vi "Transfer Offsets.vi"(1 "error in":errorcluster) -> (0 "error out":errorcluster)   [LabVIEW 2009]
uses:
  Data Access Objects/Metadata/DAO Actions.ctl
  Global Data/Dataset Transaction Id.ctl
  Global Data/Dataset Source.ctl
  Global Data/Dataset Type.ctl
  Apps/Yes No Button.ctl
  Data Access Objects/Metadata/LBCB Number.ctl
  Control Loop/LBCB_Conversions_Actions.ctl
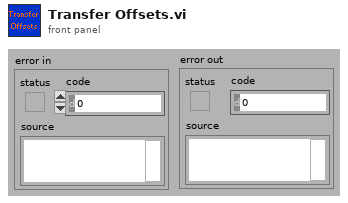
[diagram p1: front panel]
types:
  T1 = typedef "Dataset Type.ctl" = enum16{"LVDT", "Load Cell", "Actuator Command", "Servo Error", "Displacement Command", "Displacement", "Force"}
  T2 = typedef "LBCB Number.ctl" = enum16{"LBCB1", "LBCB2"}
  T3 = typedef "Dataset Source.ctl" = enum16{"LBCB 1", "LBCB 2", "Combined", "External Sensors"}
  T4 = typedef "Dataset Transaction Id.ctl" = cluster{"Dataset Source":T3, "Dataset Type":T1, "Hold":T5, "Volts":T5, "Tag":string}
  T5 = typedef "Yes No Button.ctl" = bool
  T6 = typedef "DAO Actions.ctl" = enum16{"Init", "Get", "Set"}
  T7 = typedef "LBCB Position.ctl" = cluster{"Motion Center":dbl[], "Transformation Matrix":dbl[][]}
  T8 = typedef "LBCB Settings.ctl" = cluster{"Size":T9, "Type":T10}
  T9 = typedef "LBCB Size.ctl" = enum16{"1/5th-scale LBCB", "Full-scale LBCB", "Portable LBCB"}
  T10 = typedef "LBCB Type.ctl" = enum16{"X Actuators On The Left", "X Actuators On The Right"}
  T11 = typedef "LBCB_Conversions_Actions.ctl" = enum16{"A2C", "C2A", "Set Log Filename", "Init"}
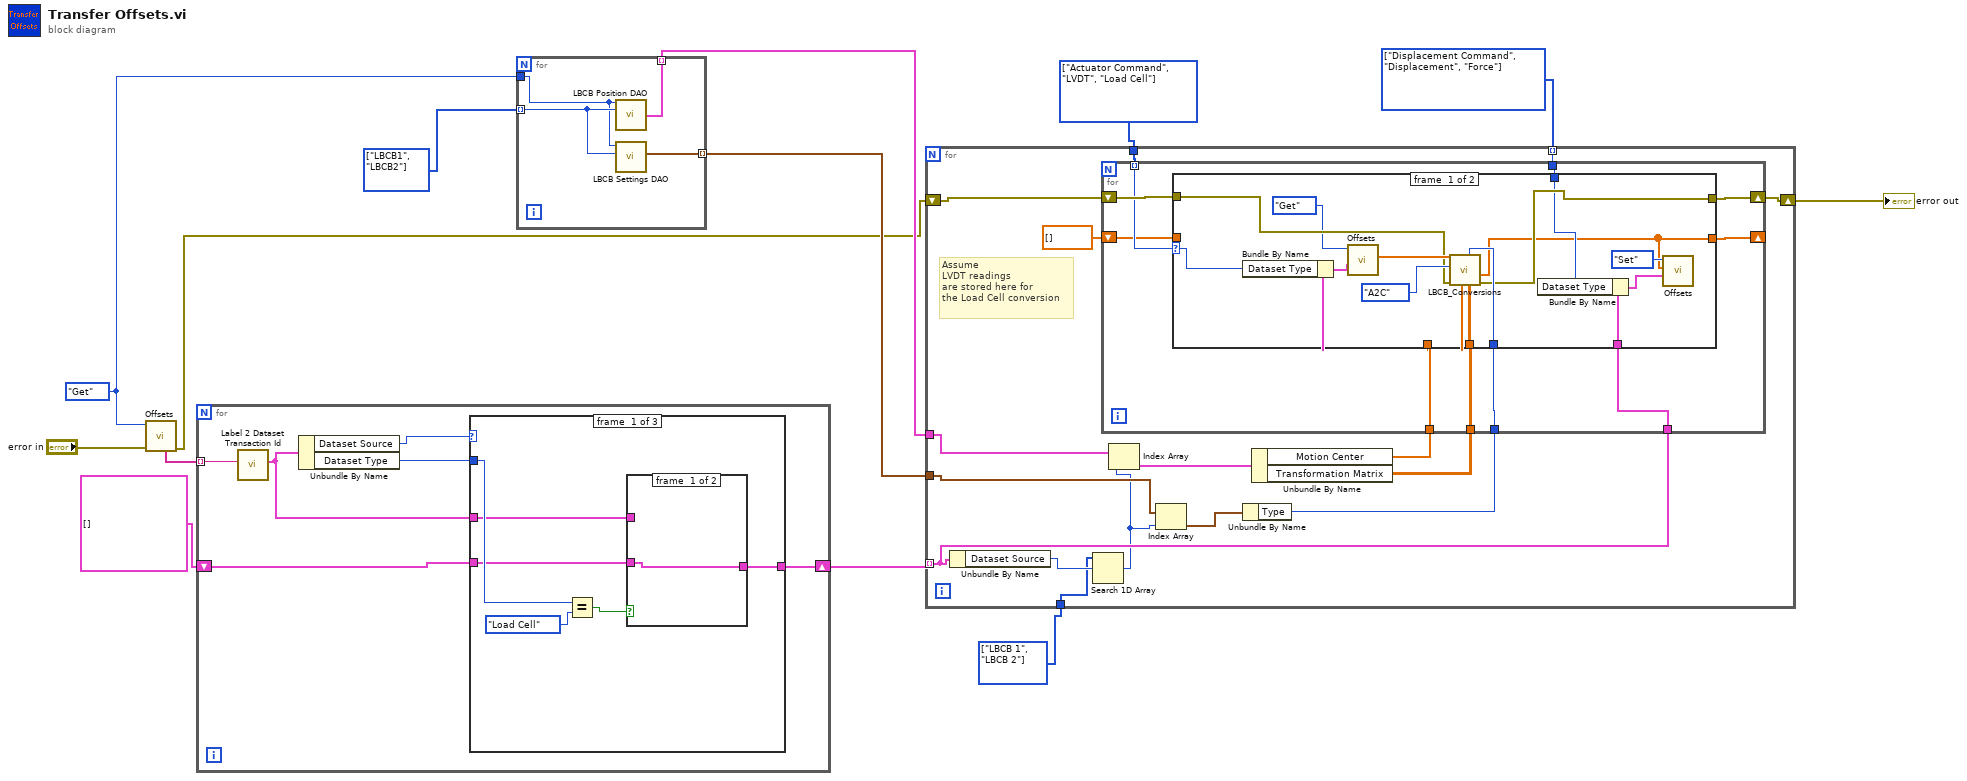
[diagram p0: block diagram]
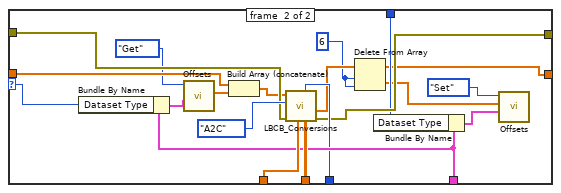
[diagram p2: hidden frame]
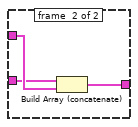
[diagram p3: hidden frame]
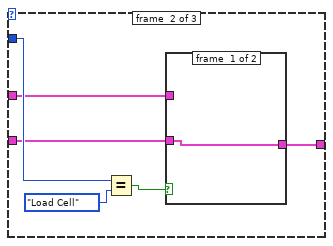
[diagram p4: hidden frame]
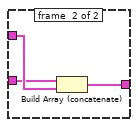
[diagram p5: hidden frame]
diagram:
  w2 = T1[] [enum."Displacement Command", enum."Displacement", enum."Force"] items=["LVDT", "Load Cell", "Actuator Command", "Servo Error", "Displacement Command", "Displacement", "Force"]
  w3 = T1[] [enum."Actuator Command", enum."LVDT", enum."Load Cell"] items=["LVDT", "Load Cell", "Actuator Command", "Servo Error", "Displacement Command", "Displacement", "Force"]
  w8 = T2[] [enum."LBCB1", enum."LBCB2"] items=["LBCB1", "LBCB2"]
  w10 = T3[] [enum."LBCB 1", enum."LBCB 2"] items=["LBCB 1", "LBCB 2", "Combined", "External Sensors"]
  w7 = DAO_Actions."Get" ("DAO Actions")
  n1 = call "Offsets.vi"("error in (no error)"="error in", "DAO Actions"=w7) -> ("error out"=w4:errorcluster, "Labels"=w12:string[])  [unwired: 7 in, 1 out]
  n2 = for {
    tunnel: w12 -> [w19] mode=indexing
    shift-right: [w15] -> w9
    shift-left: T4[] [] -> [w14]
    n3 = call "Label 2 Dataset Transaction Id.vi"("Label"=w19) -> ("Dataset Trans Id"=w16:T4)  [unwired: 10 in]
    n4 = Unbundle By Name(w16) -> ("Dataset Source"=w18:T3, "Dataset Type"=w17:T1)
    n5 = case shown="\"LBCB 2\"" w18 {
      tunnel: w17 -> [w25 w35 _]
      tunnel: w16 -> [w22 w32 _]
      tunnel: [w21 w31 w40] -> w15
      tunnel: w14 -> [w20 w30 w40]
      frame #0 {
        n6 = Equal?(x=w25, y=Dataset_Type."Load Cell") -> (x = y?=w23:bool)
        n7 = case shown="False" w23 {
          tunnel: w22 -> [_ w29]
          tunnel: [w26 w28] -> w21
          tunnel: w20 -> [w26 w27]
          frame #0 {
          }
          frame #1 {
            n8 = Build Array (concatenate)(w27, w29) -> (w28:T4[])
          }
        }
      }
      frame #1 {
        n9 = Equal?(x=w35, y=Dataset_Type."Load Cell") -> (x = y?=w33:bool)
        n10 = case shown="True" w33 {
          tunnel: w32 -> [_ w39]
          tunnel: [w36 w38] -> w31
          tunnel: w30 -> [w36 w37]
          frame #0 {
          }
          frame #1 {
            n11 = Build Array (concatenate)(w37, w39) -> (w38:T4[])
          }
        }
      }
      frame #2 {
      }
    }
  }
  n12 = for {
    tunnel: w8 -> [w44] mode=indexing
    tunnel: w7 -> [w43]
    tunnel: [w42] -> w6 mode=indexing
    tunnel: [w41] -> w5 mode=indexing
    n13 = call "LBCB Position DAO.vi"("LBCB Settings Actions"=w43, "LBCB Number"=w44) -> ("LBCB Position Output"=w42:T7)  [unwired: 11 in, 2 out]
    n14 = call "LBCB Settings DAO.vi"("LBCB Number"=w44, "Actions"=w43) -> ("LBCB Setting Out"=w41:T8)  [unwired: 7 in, 2 out]
  }
  n15 = for {
    tunnel: w9 -> [w56] mode=indexing
    tunnel: w10 -> [w54]
    tunnel: w6 -> [w60]
    tunnel: w5 -> [w59]
    shift-right: [w48] -> w1
    shift-left: w4 -> [w50]
    tunnel: w3 -> [w47]
    tunnel: w2 -> [w46] mode=indexing
    # "Assume\nLVDT readings\nare stored here for\nthe Load Cell conversion"
    n16 = Unbundle By Name(w56) -> ("Dataset Source"=w55:T3)
    n17 = Search 1D Array(1D array=w54, element=w55) -> (index of element=w51:i32)  [unwired: 1 in]
    n18 = Index Array(array=w60, index=w51) -> (element=w53:T7)
    n19 = Index Array(array=w59, index=w51) -> (element=w52:T8)
    n20 = Unbundle By Name(w52) -> ("Type"=w49:T10)
    n21 = Unbundle By Name(w53) -> ("Motion Center"=w58:dbl[], "Transformation Matrix"=w57:dbl[][])
    n22 = for {
      tunnel: w58 -> [w70]
      tunnel: w57 -> [w69]
      tunnel: w56 -> [w68]
      tunnel: w49 -> [w66]
      tunnel: w47 -> [w62] mode=indexing
      shift-right: [w65] -> w48
      shift-left: w50 -> [w67]
      tunnel: w46 -> [w64]
      shift-right: [w63] -> _
      shift-left: dbl[] [] ("Output") -> [w61]
      n23 = case shown="\"Load Cell\"" w62 {
        selector: w62 -> [w72 w92]
        tunnel: w70 -> [w83 w103]
        tunnel: w69 -> [w82 w102]
        tunnel: w68 -> [w79 w99]
        tunnel: w67 -> [w78 w98]
        tunnel: w66 -> [w77 w97]
        tunnel: [w76 w96] -> w65
        tunnel: w64 -> [w75 w95]
        tunnel: [w73 w87] -> w63
        tunnel: w61 -> [_ w90]
        frame #0 {
          n24 = Bundle By Name(cluster=w79, "Dataset Type"=w72) -> (w81:T4)
          n25 = call "Offsets.vi"("Dataset Trans Id"=w81, "DAO Actions"=DAO_Actions."Get") -> ("Data Out"=w84:dbl[])  [unwired: 7 in, 2 out]
          n26 = call "LBCB_Conversions.vi"("Transformation Matrix"=w82, "Type"=w77, "Motion Center"=w83, "error in (no error)"=w78, "Conversion Type"=LBCB_Conversions_Actions."A2C", "Input"=w84) -> ("error out"=w76:errorcluster, "Output"=w73:dbl[])  [unwired: 4 in]
          n27 = Bundle By Name(cluster=w79, "Dataset Type"=w75) -> (w80:T4)
          n28 = call "Offsets.vi"("Dataset Trans Id"=w80, "Data In"=w73, "DAO Actions"=DAO_Actions."Set") -> ()  [unwired: 6 in, 3 out]
        }
        frame #1 {
          w88 = 6 ("length")
          n29 = Bundle By Name(cluster=w99, "Dataset Type"=w92) -> (w101:T4)
          n30 = call "Offsets.vi"("Dataset Trans Id"=w101, "DAO Actions"=DAO_Actions."Get") -> ("Data Out"=w104:dbl[])  [unwired: 7 in, 2 out]
          n31 = Build Array (concatenate)(w90, w104) -> (w91:dbl[])
          n32 = call "LBCB_Conversions.vi"("Transformation Matrix"=w102, "Type"=w97, "Motion Center"=w103, "error in (no error)"=w98, "Conversion Type"=LBCB_Conversions_Actions."A2C", "Input"=w91) -> ("error out"=w96:errorcluster, "Output"=w93:dbl[])  [unwired: 4 in]
          n33 = Delete From Array(array=w93, length=w88, index=w88) -> (deleted portion=w89:dbl[], array with subset deleted=w87:dbl[])
          n34 = Bundle By Name(cluster=w99, "Dataset Type"=w95) -> (w100:T4)
          n35 = call "Offsets.vi"("Dataset Trans Id"=w100, "Data In"=w89, "DAO Actions"=DAO_Actions."Set") -> ()  [unwired: 6 in, 3 out]
        }
      }
    }
  }
  "error out" <- w1
